vi "Write ASCII Char.vi"(8 "error in (no error)":errorcluster, 9 "Char":string, 11 "HT16K33 LED Driver in":refnum<class "HT16K33 LED Driver.lvclass">) -> (0 "error out":errorcluster, 3 "HT16K33 LED Driver out":refnum<class "HT16K33 LED Driver.lvclass">)   [LabVIEW 2020, in "CTI-Peripheral.lvlib" / "HT16K33 LED Driver.lvclass"]
uses:
  HT16K33 LED Driver.lvclass
  HT16K33 LED Driver.lvclass/HT16K33 LED Driver.ctl
  CTI/I2C Connection/I2C Connection.lvclass/I2C Connection.ctl
  CTI/Session/I2C Write Data.vi
  CTI/I2C Connection/I2C Connection.lvclass
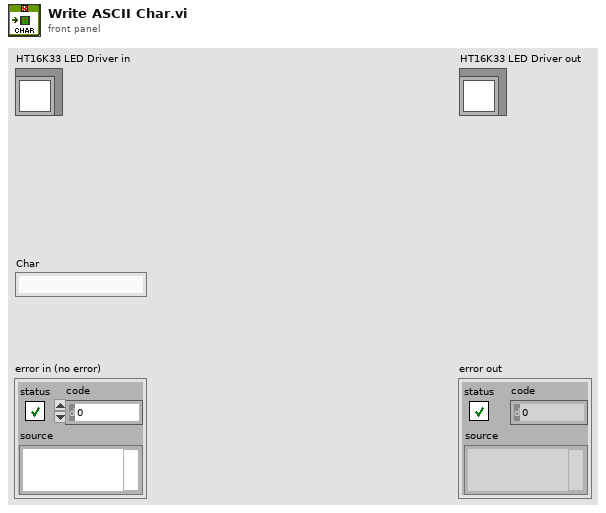
[diagram p1: front panel]
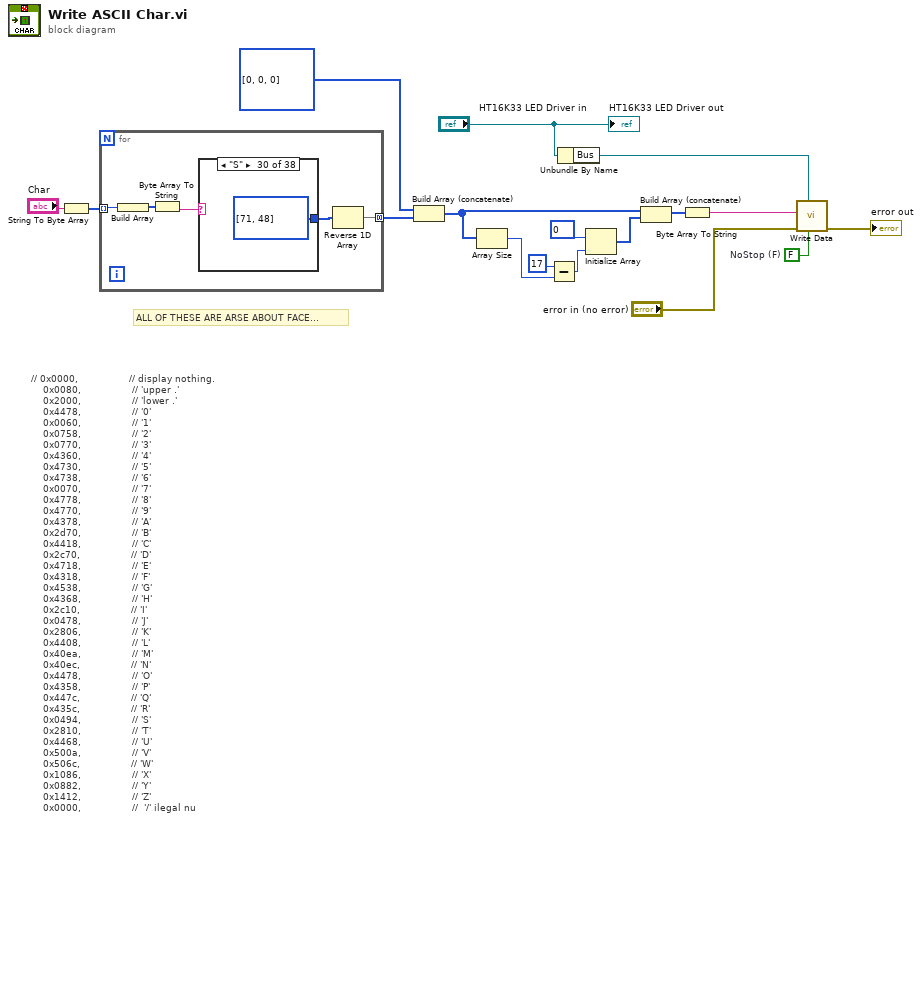
[diagram p0: block diagram]
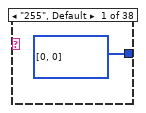
[diagram p2: hidden frame]
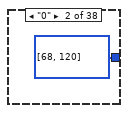
[diagram p3: hidden frame]
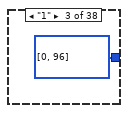
[diagram p4: hidden frame]
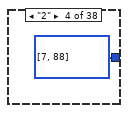
[diagram p5: hidden frame]
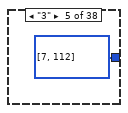
[diagram p6: hidden frame]
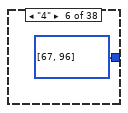
[diagram p7: hidden frame]
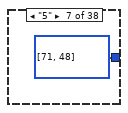
[diagram p8: hidden frame]
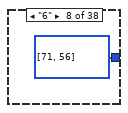
[diagram p9: hidden frame]
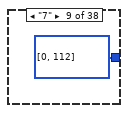
[diagram p10: hidden frame]
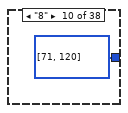
[diagram p11: hidden frame]
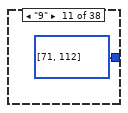
[diagram p12: hidden frame]
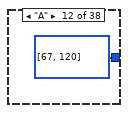
[diagram p13: hidden frame]
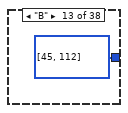
[diagram p14: hidden frame]
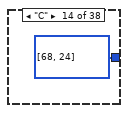
[diagram p15: hidden frame]
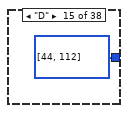
[diagram p16: hidden frame]
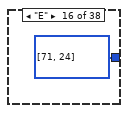
[diagram p17: hidden frame]
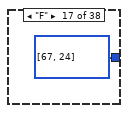
[diagram p18: hidden frame]
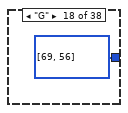
[diagram p19: hidden frame]
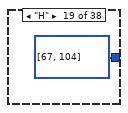
[diagram p20: hidden frame]
diagram:
  w17 = FALSE  # NoStop (F)
  # "ALL OF THESE ARE ARSE ABOUT FACE..."
  # "// 0x0000,                 // display nothing.\n    0x0080,                 // 'upper .'\n    0x2000,                 // 'lower .'\n    0x4478,                 // '0'\n    0x0060,                 // '1'\n    0x0758,                 // '2'\n    0x0770,                 // '3'\n    0x4360,                 // '4'\n    0x4730,                 // '5'\n    0x4738,                 // '6'\n    0x0070,                 // '7'\n    0x4778,                 // '8'\n    0x4770,                 // '9'\n    0x4378,                 // 'A'\n    0x2d70,                 // 'B'\n    0x4418,                 // 'C'\n    0x2c70,                 // 'D'\n    0x4718,                 // 'E'\n    0x4318,                 // 'F'\n    0x4538,                 // 'G'\n    0x4368,                 // 'H'\n    0x2c10,                 // 'I'\n    0x0478,                 // 'J'\n    0x2806,                 // 'K'\n    0x4408,                 // 'L'\n    0x40ea,                 // 'M'\n    0x40ec,                 // 'N'\n    0x4478,                 // 'O'\n    0x4358,                 // 'P'\n    0x447c,                 // 'Q'\n    0x435c,                 // 'R'\n    0x0494,                 // 'S'\n    0x2810,                 // 'T'\n    0x4468,                 // 'U'\n    0x500a,                 // 'V'\n    0x506c,                 // 'W'\n    0x1086,                 // 'X'\n    0x0882,                 // 'Y'\n    0x1412,                 // 'Z'\n    0x0000,                 //  '/' ilegal nu"
  n1 = String To Byte Array(string="Char") -> (unsigned byte array=w13:u8[])
  n2 = for {
    tunnel: w13 -> [w21] mode=indexing
    tunnel: [w18] -> w1 mode=concatenating
    n3 = Build Array(w21) -> (w20:u8[])
    n4 = Byte Array To String(unsigned byte array=w20) -> (string=w22:string)
    n5 = case shown="\"S\"" w22 {
      tunnel: [u8[] [0, 0] u8[] [68, 120] u8[] [0, 96] u8[] [7, 88] u8[] [7, 112] u8[] [67, 96] u8[] [71, 48] u8[] [71, 56] u8[] [0, 112] u8[] [71, 120] u8[] [71, 112] u8[] [67, 120] u8[] [45, 112] u8[] [68, 24] u8[] [44, 112] u8[] [71, 24] u8[] [67, 24] u8[] [69, 56] u8[] [67, 104] u8[] [44, 16] u8[] [4, 120] u8[] [40, 6] u8[] [68, 8] u8[] [64, 234] u8[] [64, 236] u8[] [68, 120] u8[] [67, 88] u8[] [68, 124] u8[] [67, 124] u8[] [71, 48] u8[] [40, 16] u8[] [68, 104] u8[] [80, 10] u8[] [80, 108] u8[] [16, 134] u8[] [8, 130] u8[] [20, 18] u8[] [32, 0]] -> w19
      frame "255", Default {
      }
      frame "0" {
      }
      frame "1" {
      }
      frame "2" {
      }
      frame "3" {
      }
      frame "4" {
      }
      frame "5" {
      }
      frame "6" {
      }
      frame "7" {
      }
      frame "8" {
      }
      frame "9" {
      }
      frame "A" {
      }
      frame "B" {
      }
      frame "C" {
      }
      frame "D" {
      }
      frame "E" {
      }
      frame "F" {
      }
      frame "G" {
      }
      frame "H" {
      }
      frame "I" {
      }
      frame "J" {
      }
      frame "K" {
      }
      frame "L" {
      }
      frame "M" {
      }
      frame "N" {
      }
      frame "O" {
      }
      frame "P" {
      }
      frame "Q" {
      }
      frame "R" {
      }
      frame "S" {
      }
      frame "T" {
      }
      frame "U" {
      }
      frame "V" {
      }
      frame "W" {
      }
      frame "X" {
      }
      frame "Y" {
      }
      frame "Z" {
      }
      frame "." {
      }
    }
    n6 = Reverse 1D Array(array=w19) -> (reversed array=w18:u8[])
  }
  n7 = Build Array (concatenate)(u8[] [0, 0, 0], w1) -> (w8:u8[])
  n8 = Array Size(array=w8) -> (size(s)=w10:i32)
  n9 = Subtract(x=17, y=w10) -> (x-y=w6:i32)
  n10 = Unbundle By Name("HT16K33 LED Driver in") -> ("Bus"=w14:refnum<class "I2C Connection.lvclass">)
  n11 = Initialize Array(u8 0, w6) -> (w5:u8[])
  n12 = Build Array (concatenate)(w8, w5) -> (w9:u8[])
  n13 = Byte Array To String(unsigned byte array=w9) -> (string=w3:string)
  n14 = call "Write Data.vi"("NoStop (F)"=w17, "I2C Connection"=w14, "error in (no error)"="error in (no error)", "Data"=w3) -> ("error out"=→"error out":errorcluster)  [unwired: 7 in]
  "HT16K33 LED Driver out" <- "HT16K33 LED Driver in"
